vi "basic_Tc-Tf.vi"() -> ()   [LabVIEW 2017]
panel:
  in  "stop":bool
  out "Tf":dbl
  in  "Tc":dbl
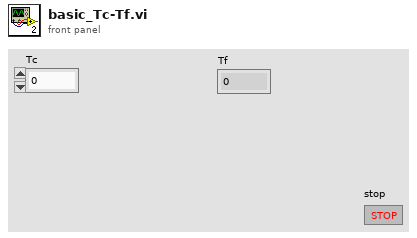
[diagram p1: front panel]
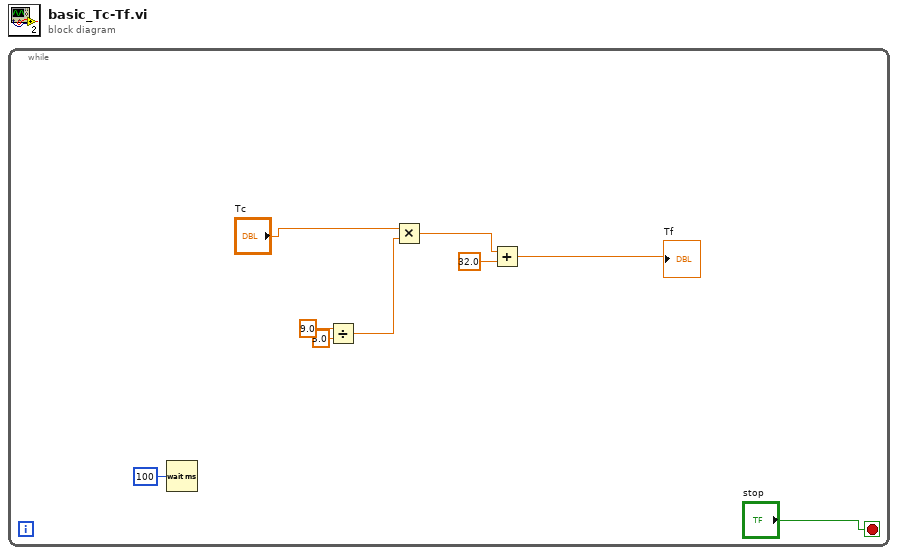
[diagram p0: block diagram]
diagram:
  n1 = while {
    stop <- "stop" stop-if-true
    n2 = Wait (ms)(milliseconds to wait=u32 100) -> ()  [unwired: 1 out]
    n3 = Divide(x=9.0, y=5.0) -> (x/y=w7:dbl)
    n4 = Multiply(x="Tc", y=w7) -> (x*y=w5:dbl)
    n5 = Add(x=w5, y=32.0) -> (x+y=→"Tf":dbl)
  }
